vi "Create Folder And Files.vi"(8 "error in (no error)":errorcluster, 11 "Config":T1 {"Hardware Configuration"."Lasers Configuration"."SettingValues"."785 Power" format="%.1f"; "Hardware Configuration"."Lasers Configuration"."SettingValues"."647 Power" format="%.1f"; "Hardware Configuration"."Lasers Configuration"."SettingValues"."561 Power" format="%.1f"}) -> (0 "error out":errorcluster, 3 "Config Out":T1 {"Hardware Configuration"."Lasers Configuration"."SettingValues"."785 Power" format="%.1f"; "Hardware Configuration"."Lasers Configuration"."SettingValues"."647 Power" format="%.1f"; "Hardware Configuration"."Lasers Configuration"."SettingValues"."561 Power" format="%.1f"})   [LabVIEW 2019, in "Logging.lvlib"]
uses:
  Logging.lvlib
  Settings/System Running Settings.ctl
  HardwareAdapter/Support/Hardware Configuration.ctl
  HardwareAdapter/Support/Camera Configuration.ctl
  C:/RM21-MMicrosopeSource/HardwareAdapter/Camera/Dependencies/PVCamNET.dll
  HardwareAdapter/Camera/Dependencies/PVCamNET.dll
  <vilib>/vision/Image Controls.llb/IMAQ Image.ctl
  C:/RM21-MMicrosopeSource/HardwareAdapter/Lasers/Dependencies/Oxxius_Boxx.dll
  HardwareAdapter/Lasers/Dependencies/Oxxius_Boxx.dll
  Logging Configuration.ctl
  Controls/DeviceStatusCtl.ctl
  Controls/CallBack Refs.ctl
  Settings/Settings.lvlib
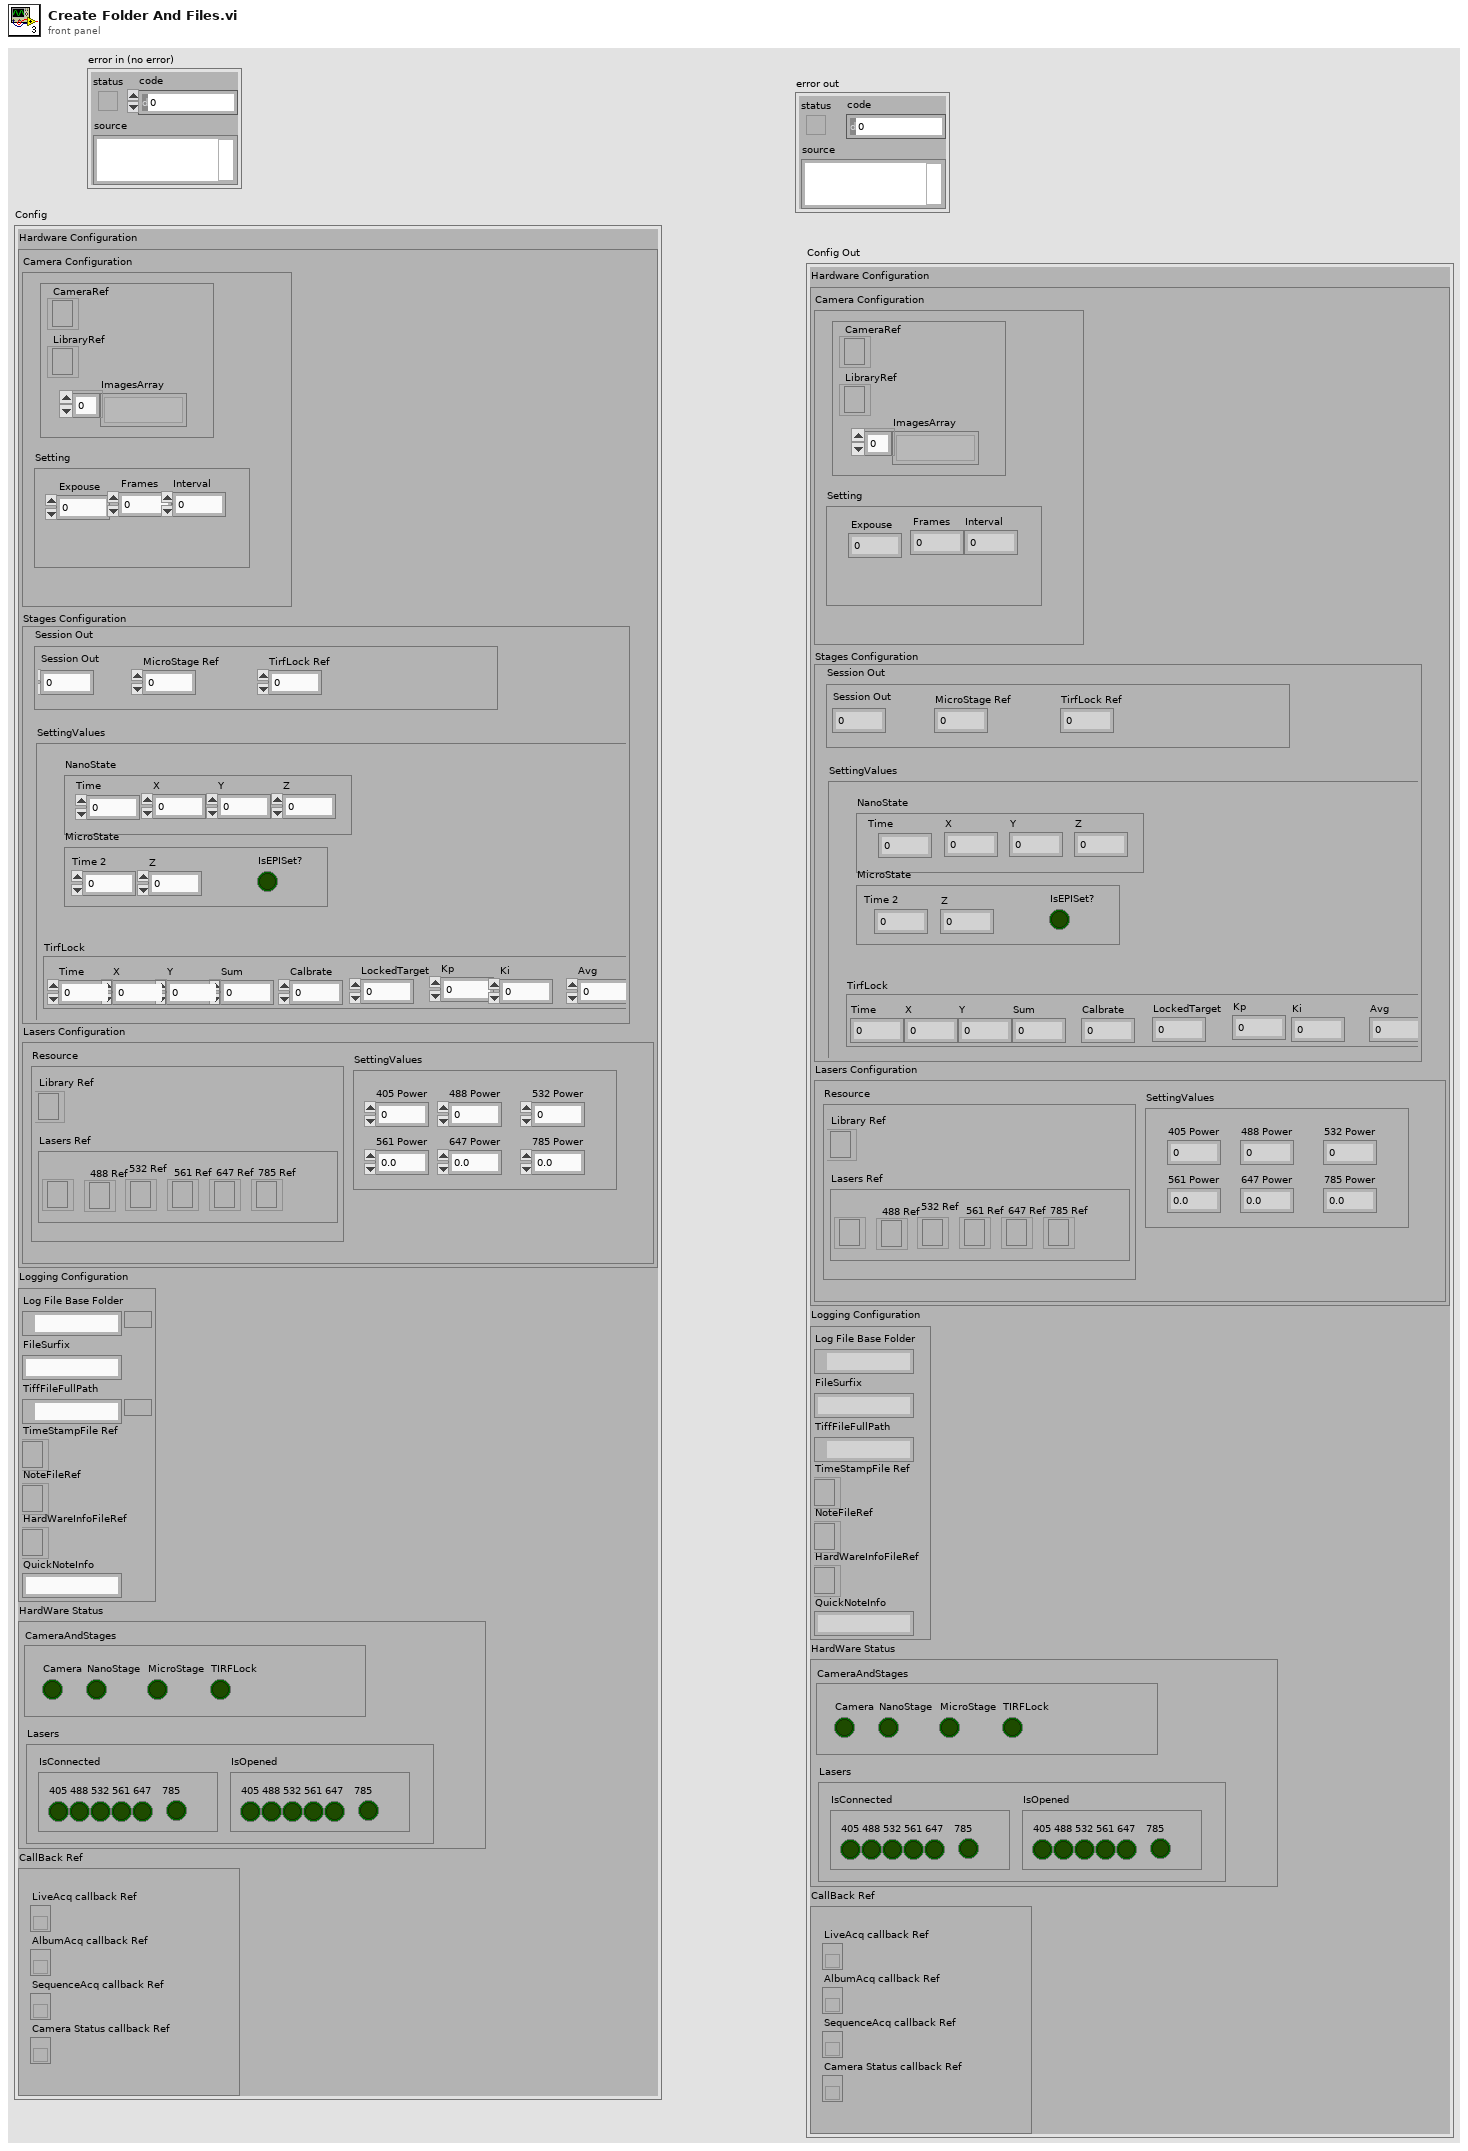
[diagram p1: front panel]
types:
  T1 = typedef "Settings.lvlib/System Running Settings.ctl" = cluster{"Hardware Configuration":T2, "Logging Configuration":T5, "HardWare Status":cluster{"CameraAndStages":T6, "Lasers":cluster{"IsConnected":cluster{"405":bool, "488":bool, "532":bool, "561":bool, "647":bool, "785":bool}, "IsOpened":cluster{"405":bool, "488":bool, "532":bool, "561":bool, "647":bool, "785":bool}}}, "CallBack Ref":T7}
  T2 = typedef "Hardware Configuration.ctl" = cluster{"Camera Configuration":T3, "Stages Configuration":cluster{"Resource":cluster{"NanoStage Ref":i32, "MicroStage Ref":i32, "TirfLock Ref":i32}, "SettingValues":cluster{"NanoState":cluster{"Time":dbl, "X":dbl, "Y":dbl, "Z":dbl}, "MicroState":cluster{"Time 2":dbl, "Z":dbl, "IsEPISet?":bool}, "TirfLock":cluster{"Time":dbl, "X":dbl, "Y":dbl, "Sum":dbl, "Calbrate":dbl, "LockedTarget":dbl, "Kp":dbl, "Ki":dbl, "Avg":dbl}}}, "Lasers Configuration":cluster{"SettingValues":cluster{"405 Power":sgl, "488 Power":sgl, "532 Power":sgl, "561 Power":sgl, "647 Power":sgl, "785 Power":sgl}, "Resource":cluster{"Library Ref":refnum<k24>, "Lasers Ref":cluster{"405 Ref":refnum<k24>, "488 Ref":refnum<k24>, "532 Ref":refnum<k24>, "561 Ref":refnum<k24>, "647 Ref":refnum<k24>, "785 Ref":refnum<k24>}}}}
  T3 = typedef "Camera Configuration.ctl" = cluster{"Setting":cluster{"Expouse":dbl, "Frames":dbl, "Interval":dbl}, "Resource":cluster{"CameraRef":refnum<k24>, "LibraryRef":refnum<k24>, "ImagesArray":T4[]}}
  T4 = typedef "IMAQ Image.ctl" = refnum<image>
  T5 = typedef "Logging.lvlib/Logging Configuration.ctl" = cluster{"Log File Base Folder":path, "FileSurfix":string, "TiffFileFullPath":path, "TimeStampFile Ref":refnum<file>, "NoteFileRef":refnum<file>, "HardWareInfoFileRef":refnum<file>, "QuickNoteInfo":string}
  T6 = typedef "DeviceStatusCtl.ctl" = cluster{"Camera":bool, "NanoStage":bool, "MicroStage":bool, "TIRFLock":bool}
  T7 = typedef "CallBack Refs.ctl" = cluster{"LiveAcq callback Ref":refnum<k27>, "AlbumAcq callback Ref":refnum<k27>, "SequenceAcq callback Ref":refnum<k27>, "Camera Status callback Ref":refnum<k27>}
  T8 = enum16{"open", "replace", "create", "open or create", "replace or create", "replace or create with confirmation"}
  T9 = cluster{"Expouse":dbl, "Frames":dbl, "Interval":dbl}
  T10 = cluster{"405 Power":sgl, "488 Power":sgl, "532 Power":sgl, "561 Power":sgl, "647 Power":sgl, "785 Power":sgl}
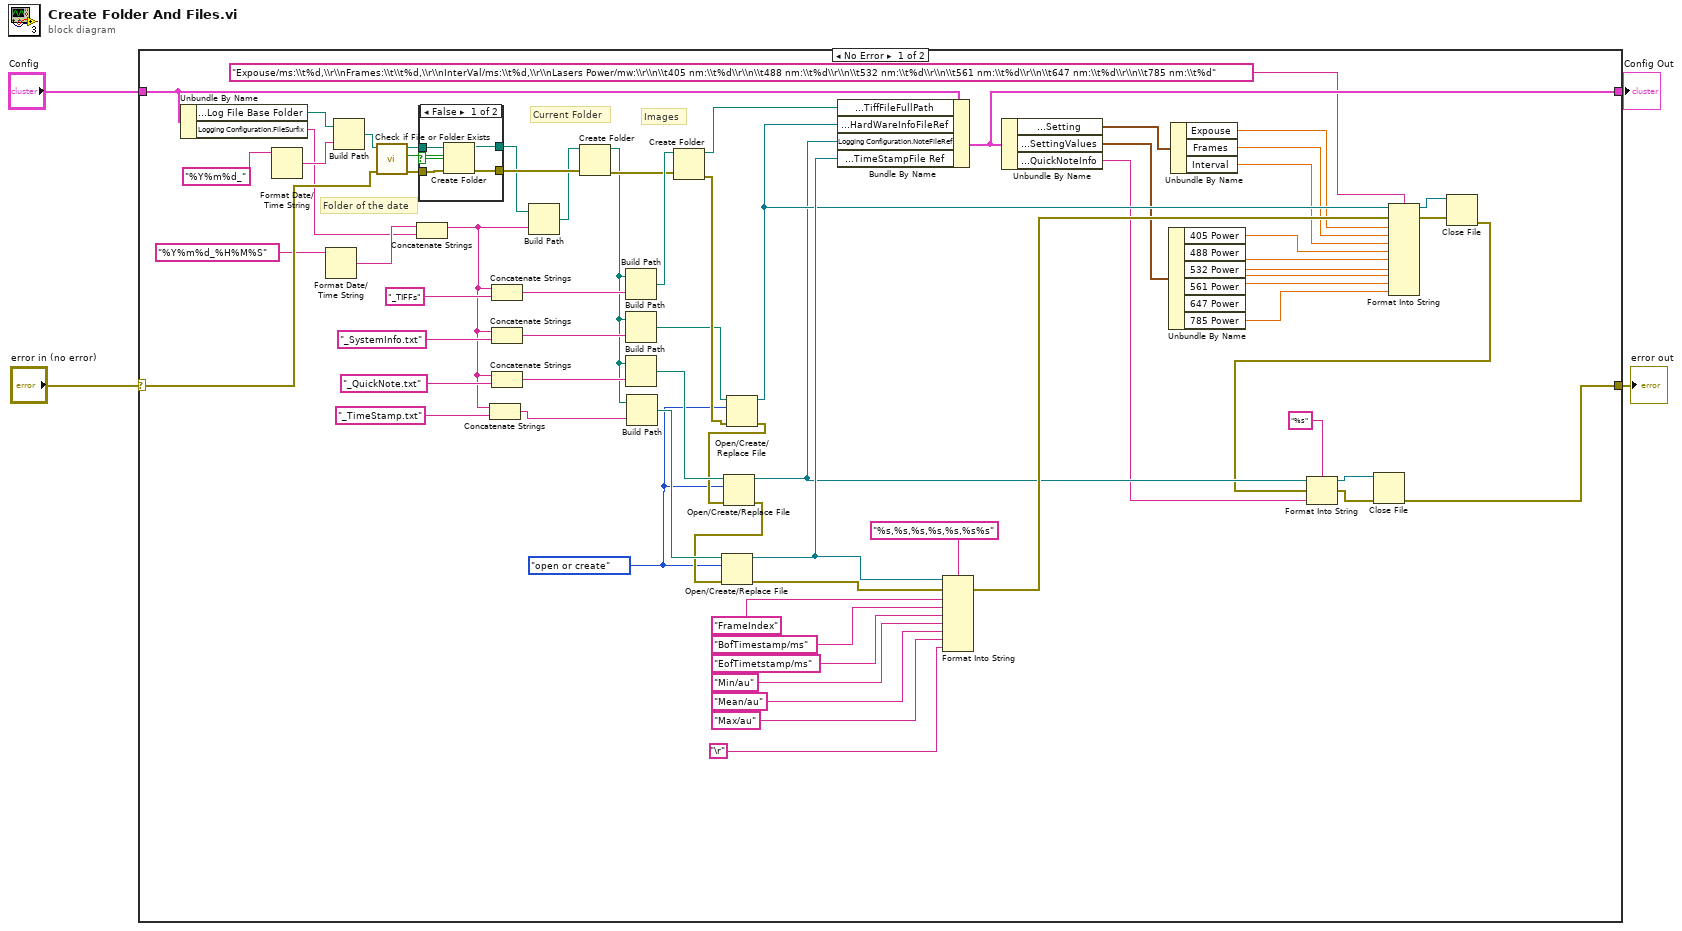
[diagram p0: block diagram]
diagram:
  n1 = case shown="No Error" "error in (no error)" {
    selector: "error in (no error)" -> [w64 w80]
    tunnel: "Config" -> [w67 w81]
    tunnel: [w26 w81] -> w2
    tunnel: [w7 w80] -> w1
    frame No Error {
      w32 = T8."open or create" ("operation (0:open)")
      # "Images"
      # "Current Folder"
      # "Folder of the date"
      n2 = Unbundle By Name(w67) -> ("Logging Configuration.Log File Base Folder"=w62:path, "Logging Configuration.FileSurfix"=w5:string)
      n3 = Format Date/Time String(time format string (%c)="%Y%m%d_") -> (date/time string=w72:string)  [unwired: 2 in]
      n4 = Format Date/Time String(time format string (%c)="%Y%m%d_%H%M%S") -> (date/time string=w6:string)  [unwired: 2 in]
      n5 = Build Path(base path=w62, name or relative path=w72) -> (appended path=w71:path)
      n6 = call <vilib>:"Check if File or Folder Exists.vi"("error in (no error)"=w64, "path"=w71) -> ("error out"=w63:errorcluster, "file or folder exists?"=w70:bool, "dup path"=w69:path)  [unwired: 7 in]
      n7 = Concatenate Strings(w6, w5) -> (w50:string)
      n8 = case shown="False" w70 {
        tunnel: w69 -> [w77 w79]
        tunnel: [w76 w78] -> w59
        tunnel: [w75 w79] -> w57
        tunnel: w63 -> [w74 w78]
        frame False {
          n9 = Create Folder(path (use dialog)=w77, error in=w74) -> (created path=w75:path, error out=w76:errorcluster)  [unwired: 1 in, 1 out]
        }
        frame True {
        }
      }
      n10 = Concatenate Strings(w50, "_TimeStamp.txt" ("string")) -> (w49:string)
      n11 = Concatenate Strings(w50, "_TIFFs" ("string")) -> (w68:string)
      n12 = Concatenate Strings(w50, "_SystemInfo.txt" ("string")) -> (w66:string)
      n13 = Concatenate Strings(w50, "_QuickNote.txt" ("string")) -> (w65:string)
      n14 = Build Path(base path=w57, name or relative path=w50) -> (appended path=w56:path)
      n15 = Create Folder(path (use dialog)=w56, error in=w59) -> (created path=w48:path, error out=w58:errorcluster)  [unwired: 1 in, 1 out]
      n16 = Build Path(base path=w48, name or relative path=w68) -> (appended path=w61:path)
      n17 = Build Path(base path=w48, name or relative path=w66) -> (appended path=w31:path)
      n18 = Build Path(base path=w48, name or relative path=w65) -> (appended path=w46:path)
      n19 = Build Path(base path=w48, name or relative path=w49) -> (appended path=w47:path)
      n20 = Create Folder(path (use dialog)=w61, error in=w58) -> (created path=w60:path, error out=w34:errorcluster)  [unwired: 1 in, 1 out]
      n21 = Open/Create/Replace File(file path (use dialog)=w31, error in=w34, operation (0:open)=w32) -> (refnum out=w29:refnum<file>, error out=w33:errorcluster)  [unwired: 3 in, 1 out]
      n22 = Open/Create/Replace File(file path (use dialog)=w46, error in=w33, operation (0:open)=w32) -> (refnum out=w28:refnum<file>, error out=w45:errorcluster)  [unwired: 3 in, 1 out]
      n23 = Open/Create/Replace File(file path (use dialog)=w47, error in=w45, operation (0:open)=w32) -> (refnum out=w39:refnum<file>, error out=w40:errorcluster)  [unwired: 3 in, 1 out]
      n24 = Bundle By Name(cluster=w67, "Logging Configuration.TiffFileFullPath"=w60, "Logging Configuration.HardWareInfoFileRef"=w29, "Logging Configuration.NoteFileRef"=w28, "Logging Configuration.TimeStampFile Ref"=w39) -> (w26:T1)
      n25 = Format Into String(format string="%s,%s,%s,%s,%s,%s%s", initial string=w39, error in=w40, "FrameIndex" ("input 1"), "BofTimestamp/ms" ("input 2"), "EofTimetstamp/ms" ("input 3"), "Min/au" ("input 1"), "Mean/au" ("input 2"), "Max/au" ("input 3"), "\r") -> (error out=w30:errorcluster)  [unwired: 1 out]
      n26 = Unbundle By Name(w26) -> ("Hardware Configuration.Camera Configuration.Setting"=w25:T9, "Hardware Configuration.Lasers Configuration.SettingValues"=w24:T10, "Logging Configuration.QuickNoteInfo"=w13:string)
      n27 = Unbundle By Name(w24) -> ("405 Power"=w19:sgl, "488 Power"=w18:sgl, "532 Power"=w17:sgl, "561 Power"=w16:sgl, "647 Power"=w15:sgl, "785 Power"=w14:sgl)
      n28 = Unbundle By Name(w25) -> ("Expouse"=w22:dbl, "Frames"=w21:dbl, "Interval"=w20:dbl)
      n29 = Format Into String(format string="Expouse/ms:\\t%d,\\r\\nFrames:\\t\\t%d,\\r\\nInterVal/ms:\\t%d,\\r\\nLasers Power/mw:\\r\\n\\t405 nm:\\t%d\\r\\n\\t488 nm:\\t%d\\r\\n\\t532 nm:\\t%d\\r\\n\\t561 nm:\\t%d\\r\\n\\t647 nm:\\t%d\\r\\n\\t785 nm:\\t%d", initial string=w29, error in=w30, w22, w21, w20, w19, w18, w17, w16, w15, w14) -> (resulting string=w10:refnum<file>, error out=w9:errorcluster)
      n30 = Close File(refnum=w10, error in=w9) -> (error out=w8:errorcluster)  [unwired: 1 out]
      n31 = Format Into String(format string="%s", initial string=w28, error in=w8, w13) -> (resulting string=w12:refnum<file>, error out=w11:errorcluster)
      n32 = Close File(refnum=w12, error in=w11) -> (error out=w7:errorcluster)  [unwired: 1 out]
    }
    frame Error {
    }
  }
  "Config Out" <- w2
  "error out" <- w1
